vi "Decode.vi"(8 "error in (no error)":errorcluster, 10 "Binary string in":string, 11 "obj in":refnum<class "Decode_Packet.lvclass">) -> (0 "error out":errorcluster, 1 "Data out":refnum<class "Data.lvclass">, 2 "Rest of binary string":string, 3 "obj out":refnum<class "Decode_Packet.lvclass">)   [LabVIEW 2020, in "Decode_Packet.lvclass"]
uses:
  Decode_Packet.lvclass
  Data Class/Data.lvclass
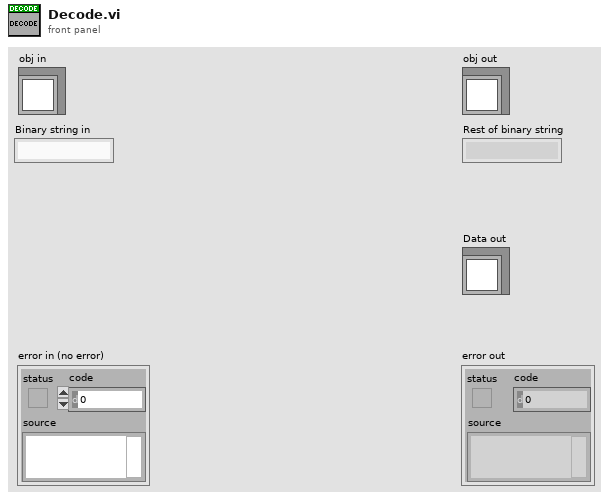
[diagram p1: front panel]
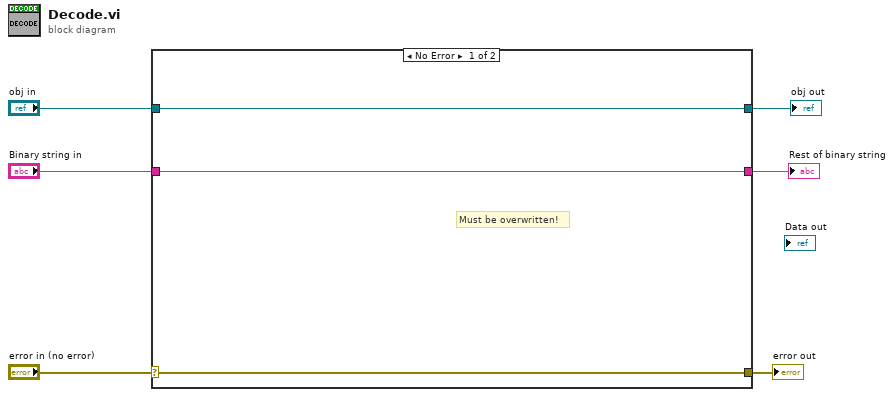
[diagram p0: block diagram]
diagram:
  n1 = case shown="No Error" "error in (no error)" {
    selector: "error in (no error)" -> [w8 w12]
    tunnel: [w8 w12] -> w5
    tunnel: [w9 w11] -> w3
    tunnel: "obj in" -> [w9 w11]
    tunnel: [w7 w10] -> w2
    tunnel: "Binary string in" -> [w7 w10]
    frame No Error {
      # "Must be overwritten!"
    }
    frame Error {
    }
  }
  "error out" <- w5
  "obj out" <- w3
  "Rest of binary string" <- w2
